vi "wrap.DestroyGLue.vi"(0 "class.GLue in":refnum<class "class.GLue.lvclass">, 11 "error in (no error)":errorcluster) -> (4 "class.GLue out":refnum<class "class.GLue.lvclass">, 15 "error out":errorcluster)   [LabVIEW 2014, in "GLue.lvlib" / "class.GLue.lvclass"]
uses:
  class.GLue.lvclass
  class.GLue.lvclass/class.GLue.ctl
  Resources/GLue.dll
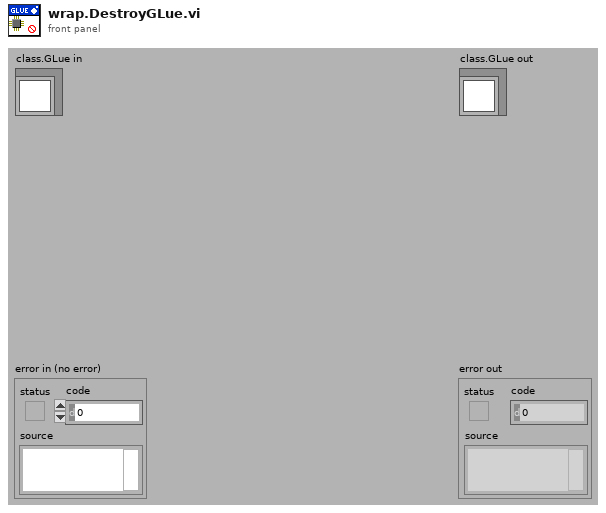
[diagram p1: front panel]
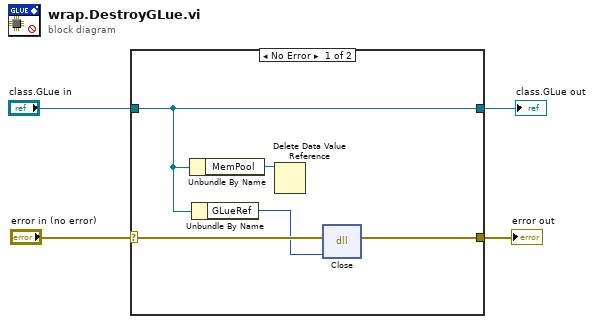
[diagram p0: block diagram]
diagram:
  n1 = case shown="No Error" "error in (no error)" {
    selector: "error in (no error)" -> [w9 w11]
    tunnel: [w8 w11] -> w3
    tunnel: [w6 w10] -> w1
    tunnel: "class.GLue in" -> [w6 w10]
    frame No Error {
      n2 = Unbundle By Name(w6) -> ("MemPool"=w5:refnum<data-value>)
      n3 = Unbundle By Name(w6) -> ("GLueRef"=w7:i64)
      n4 = Delete Data Value Reference(data value reference=w5) -> ()  [unwired: 1 in, 2 out]
      n5 = dll-call lib="C:/Users/Antonie/Documents/work/glue/trunk/Resources/GLue.dll" fn="Close"(error in=w9, "MLua"=w7) -> (error out=w8:errorcluster)  [unwired: 4 in, 1 out]
    }
    frame Error {
    }
  }
  "error out" <- w3
  "class.GLue out" <- w1
